vi "spring - delete item.vi"(7 "tree ref":refnum<vi>, 8 "error in (no error)":errorcluster, 11 "tag":string) -> (0 "error out":errorcluster)   [LabVIEW 2014]
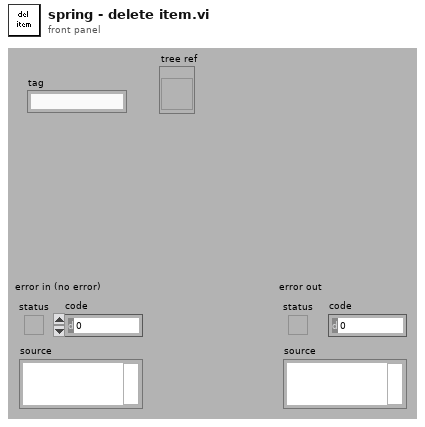
[diagram p1: front panel]
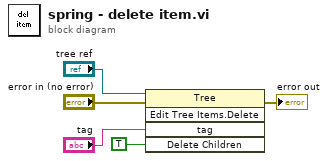
[diagram p0: block diagram]
diagram:
  n1 = invoke class="Tree" method="Edit Tree Items.Delete"(reference="tree ref", error in="error in (no error)", "tag"="tag", "Delete Children"=TRUE) -> (error out=→"error out":errorcluster)  [unwired: 1 in, 4 out]
